vi "Join String Array.vi"(11 "Array":string[](array[string])) -> (3 "String":string)   [LabVIEW 2015]
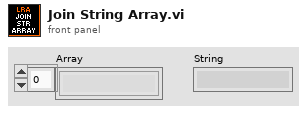
[diagram p1: front panel]
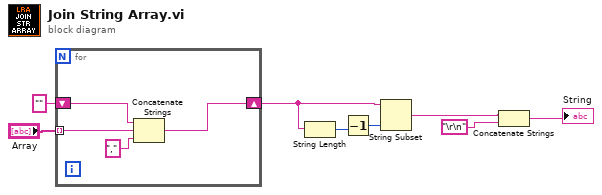
[diagram p0: block diagram]
diagram:
  n1 = for {
    tunnel: "Array" -> [w12] mode=indexing
    shift-right: [w10] -> w5
    shift-left: "" -> [w9]
    n2 = Concatenate Strings(w9, w12, "," ("string")) -> (w10:string)
  }
  n3 = String Length(string=w5) -> (length=w6:i32)
  n4 = Decrement(x=w6) -> (x-1=w7:i32)
  n5 = String Subset(string=w5, length (rest)=w7) -> (substring=w3:string)  [unwired: 1 in]
  n6 = Concatenate Strings(w3, "\r\n") -> (→"String":string)
